vi "Create Class ObjectData DVR.vi"(8 "error in (no error)":errorcluster, 11 "Main in":refnum<class "Main.lvclass">) -> (0 "error out":errorcluster, 3 "Main out":refnum<class "Main.lvclass">)   [LabVIEW 2019, in "Main.lvclass"]
doc: "Developed by Kevin Thompson\nkevin@thompsonengineering.net\n\nCopyright 2018\nThompson Engineering, LLC"
uses:
  Main.lvclass
  DataTypes/ObjData--cluster.ctl
  DataTypes/Settings--cluster.ctl
  support/Data Algorithms/subvis/DataTypes/Gain control.ctl
  support/Data Algorithms/subvis/DataTypes/ESR scaling--cluster.ctl
  DataTypes/Public Events--cluster.ctl
  Common/DataTypes/TD Async CmdMsg EventData--cluster.ctl
  Common/DataTypes/UpdateControlValue EvData--cluster.ctl
  DataTypes/ProcessingStateChg EvData--cluster.ctl
  DataTypes/ProcessingState--enum.ctl
  DataTypes/Dependency--cluster.ctl
  Config/Config.lvclass
  DAQ_Engine/DAQ_Engine.lvclass
  Log_Engine/Log_Engine.lvclass
  DataTypes/Read Data--cluster.ctl
  Common/DataTypes/InverterWaveforms--QRef.ctl
  Common/DataTypes/InverterWaveforms--cluster.ctl
  Common/DataTypes/ChannelWaveforms--cluster.ctl
  Common/DataTypes/RawDAQDataQRef--cluster.ctl
  Common/DataTypes/RawDAQData--cluster.ctl
  Common/DataTypes/RawChannelData--cluster.ctl
  Common/DataTypes/Measurement Config--cluster.ctl
  Common/DataTypes/Acquisition Mode--cluster.ctl
  DAQ_Engine/DataTypes/DAQStateEvData--cluster.ctl
  Common/DataTypes/DAQState--enum.ctl
  DataTypes/Private Events--cluster.ctl
  Common/DataTypes/DataProcAuxDat--Qref.ctl
  DataTypes/DataProcessAuxData--cluster.ctl
  DataTypes/InverterInfo--cluster.ctl
  Common/DataTypes/Inverter database record v2--cluster.ctl
  Common/DataTypes/inverter info v2--cluster.ctl
  Common/DataTypes/inverter gain range--cluster.ctl
  Common/DataTypes/inverter offset range--cluster.ctl
  <vilib>/TELLC/Dynamic CVT API/TD Dynamic CVT DVR--ref.ctl
  Main.lvclass/Main.ctl
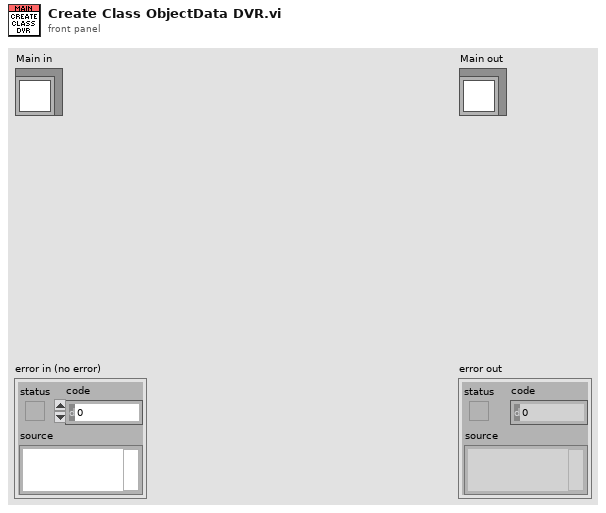
[diagram p1: front panel]
types:
  T1 = typedef "Main.lvclass/ObjData--cluster.ctl" = cluster{"Settings":T2, "Public Events":T5, "Dependency":T6, "ReadData-placeholder":T7, "VISA-placeholder":refnum<visa-resource-name>, "InverterWaveformsQ":T8, "Application.TerminateProcess Event":refnum<user-event>, "RawDaqDataQ":T9, "MeasSettings":T10, "InverterDataAcqMode":T11, "DAQState Data":T12, "Private Events":T14, "InvWfmsQ-DT":T8, "DPAuxDataQ":T15, "ProcessingState":T16, "InverterInfo":T17, "CurrInverters":T18[], "InverterLUT Dict":T22, "ESR Chart Ref":refnum<vi>[], "StoreESR BLine Ref":refnum<vi>, "UseSavedESR BLine Ref":refnum<vi>}
  T2 = typedef "Main.lvclass/Settings--cluster.ctl" = cluster{"Simulation":bool, "Signal scaling":T3[], "ESR scaling":T4[], "num readings to average":i32[], "ESR alarm threshhold (%)":i32[], "UseDummyVrms":bool, "Dummy Vrms":dbl, "Inverter Database File":path, "default Inverter (name)":string[]}
  T3 = typedef "Main.lvclass/Gain control.ctl" = cluster{"Iin ripple gain":dbl, "Iout ripple gain":dbl, "Iout 60Hz gain ":dbl, "Vout 60Hz gain ":dbl, "Iin ripple offest":dbl, "Iout ripple offset":dbl, "Iout 60Hz offset":dbl, "Vout 60Hz offset":dbl}
  T4 = typedef "Main.lvclass/ESR scaling--cluster.ctl" = cluster{"Gain":dbl, "Offset":dbl}
  T5 = typedef "Main.lvclass/Public Events--cluster.ctl" = cluster{"Main.AsyncCmd Event":refnum<user-event>, "Main.AsyncMsg Event":refnum<user-event>, "stop process":refnum<user-event>, "UpdateControlValue Ev":refnum<user-event>, "ProcessingStateChg Ev":refnum<user-event>}
  T6 = typedef "Main.lvclass/Dependency--cluster.ctl" = cluster{"Config":refnum<class "Config.lvclass">, "DAQ":refnum<class "DAQ_Engine.lvclass">, "Log_Engine":refnum<class "Log_Engine.lvclass">}
  T7 = typedef "Main.lvclass/Read Data--cluster.ctl" = cluster{"Data":dbl}
  T8 = typedef "InverterWaveforms--QRef.ctl" = refnum<queue>
  T9 = typedef "RawDAQDataQRef--cluster.ctl" = refnum<queue>
  T10 = typedef "Measurement Config--cluster.ctl" = cluster{"Data Rate 9775":dbl, "Data Rate 9215":dbl, "Samples RMS 9215":u32, "Samples RMS 9775":u32}
  T11 = typedef "Acquisition Mode--cluster.ctl" = enum16{"3phase", "Single"}
  T12 = typedef "DAQ_Engine.lvclass/DAQStateEvData--cluster.ctl" = cluster{"DAQState":T13, "vData":variant}
  T13 = typedef "DAQState--enum.ctl" = enum16{"Unknown", "Stopped", "Running", "Error"}
  T14 = typedef "Main.lvclass/Private Events--cluster.ctl" = cluster{"PrivateAsync Ev":refnum<user-event>}
  T15 = typedef "DataProcAuxDat--Qref.ctl" = refnum<queue>
  T16 = typedef "Main.lvclass/ProcessingState--enum.ctl" = enum16{"Idle", "Starting", "Running", "Done", "Error"}
  T17 = typedef "InverterInfo--cluster.ctl" = cluster{"Inverter ID":string}
  T18 = typedef "Inverter database record v2--cluster.ctl" = cluster{"name":string, "last updated":timestamp, "type":string, "inverter Info":T19, "gain range":T20, "offset range":T21, "gain actual":dbl, "offset actual":dbl, "power level":dbl, "minimum current":dbl, "resistance single phase":dbl, "resistance 3 phase":dbl, "set flag":u16}
  T19 = typedef "inverter info v2--cluster.ctl" = cluster{"manufacturer":string, "model":string, "product":string, "serial":string, "power class":string, "year manf":string}
  T20 = typedef "inverter gain range--cluster.ctl" = cluster{"gain max":dbl, "gain min":dbl, "gain increment":dbl}
  T21 = typedef "inverter offset range--cluster.ctl" = cluster{"offset max":dbl, "offset min":dbl, "offset increment":dbl}
  T22 = typedef "TD Dynamic CVT DVR--ref.ctl" = refnum<data-value>
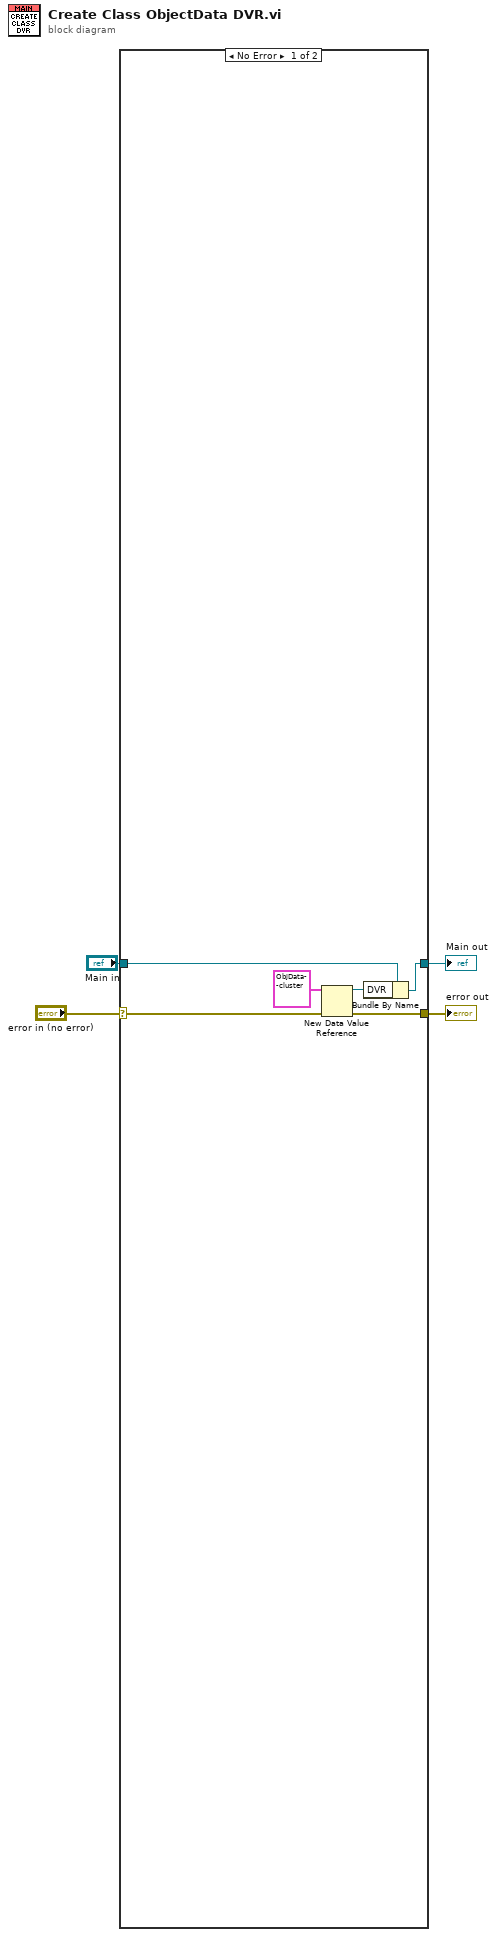
[diagram p0: block diagram]
diagram:
  n1 = case shown="No Error" "error in (no error)" {
    selector: "error in (no error)" -> [w9 w12]
    tunnel: [w8 w12] -> w3
    tunnel: [w6 w11] -> w1
    tunnel: "Main in" -> [w7 w11]
    frame No Error {
      n2 = New Data Value Reference(data value=T1 {"Settings"={"Simulation"=FALSE, "Signal scaling"=[], "ESR scaling"=[], "num readings to average"=[], "ESR alarm threshhold (%)"=[], "UseDummyVrms"=FALSE, "Dummy Vrms"=0.0, "Inverter Database File"=path "", "default Inverter (name)"=[]}, "Public Events"={"Main.AsyncCmd Event"=refnum, "Main.AsyncMsg Event"=refnum, "stop process"=refnum, "UpdateControlValue Ev"=refnum, "ProcessingStateChg Ev"=refnum}, "Dependency"={"Config"=refnum, "DAQ"=refnum, "Log_Engine"=refnum}, "ReadData-placeholder"={"Data"=0.0}, "VISA-placeholder"="", "InverterWaveformsQ"=refnum, "Application.TerminateProcess Event"=refnum, "RawDaqDataQ"=refnum, "MeasSettings"={"Data Rate 9775"=0.0, "Data Rate 9215"=0.0, "Samples RMS 9215"=0, "Samples RMS 9775"=0}, "InverterDataAcqMode"=enum."3phase", "DAQState Data"={"DAQState"=enum."Unknown", "vData"=variant}, "Private Events"={"PrivateAsync Ev"=refnum}, "InvWfmsQ-DT"=refnum, "DPAuxDataQ"=refnum, "ProcessingState"=enum."Idle", "InverterInfo"={"Inverter ID"=""}, "CurrInverters"=[], "InverterLUT Dict"=refnum, "ESR Chart Ref"=[], "StoreESR BLine Ref"=refnum, "UseSavedESR BLine Ref"=refnum} ("ObjData"), error in=w9) -> (data value reference=w10:refnum<data-value>, error out=w8:errorcluster)
      n3 = Bundle By Name(cluster=w7, "DVR"=w10) -> (w6:refnum<class "Main.lvclass">)
    }
    frame Error {
    }
  }
  "error out" <- w3
  "Main out" <- w1
